vi "FOV_Zoom_Frame to Hex.vi"(8 "Objective":i8=20, 9 "Z pixel Size":i8=4, 11 "AOL_Globals":T1={"Imaging Protocol"=enum."AOL Z-Stack", "Number of POI"=0, "Number of Miniscans"=0, "Number of Trials"=0, "Number of Cycles "=0, "# Averaged Frames"=0, "Laser power (%)"=0, "Pockels (V)"=0.0, "Acquisition Length (sec)"=0.0, "Fill time (us)"=0.0, "POI Dwell time (us)"=0.0, "Miniscan Dwell time per pixel (us)"=0.0, "PMT 1"=0.0, "PMT 2"=0.0, "Back Apperture (mA)"=0.0, "Frame Size"=0, "Center Frequency"=0.0, "Field of View (norm)"=0.0, "DwellTime (us)"=0.0, "Wavelength (nm)"=0.0, "Zoom"=0.0, "AOL Z"=0.0, "AOL Mode"=enum."Raster", "GridXY"=0.0, "GridZ"=0.0, "TriggerPeriod (sec)"=0.0, "Number of Pixels in Miniscan"=0, "Experiment folder path"=path "", "X centre"=0.0, "Y centre"=0.0, "Angle (degrees)"=0.0, "Plane Mode"=0, "Threshold"=[], "Regenerate Chirps"=FALSE, "Rectangle ROI length (pixels)"=0, "Rectangle ROI height (pixels)"=0, "AOD fill"=4900, "StartupDelay"=0, "Samples Wait after Trigger"=5080, "Slip Cycle"=600000, "Add Cycle"=TRUE, "Functional Mode"=enum."Point", "Z Start"=0.0, "Z Stop"=0.0, "# Planes"=0} {"Plane Mode" items=["XY Plane", "XZ Plane", "YZ Plane", "arbitraryplane"]; "Frame Size" items=["100X100"=100, "128X128"=128, "200X200"=200, "256X256"=256, "512X512"=512, "1024x1024"=1024, "2048x2048"=2048]; "Back Apperture (mA)" format="%#.6g"; "Pockels (V)" format="%#.6g"; "PMT 2" format="%#.6g"; "PMT 1" format="%#.6g"; "Angle (degrees)" format="%#.6g"; "POI Dwell time (us)" format="%#.6g"}) -> (3 "FOV-Zoom-FrameSize Hex":string)   [LabVIEW 2017]
uses:
  Typedefs/Controls/AOL_Globals.ctl
  Typedefs/Imaging Protocols enum.ctl
  Typedefs/Frame Size.ctl
  Typedefs/AOL modes.ctl
  Typedefs/Plane Mode.ctl
  Typedefs/Functional Mode.ctl
  <vilib>/Utility/miscctls.llb/LVStringsAndValuesArrayTypeDef_SGL.ctl
panel:
  out "Field of view (um)":dbl
  # "SUBROUTINE"
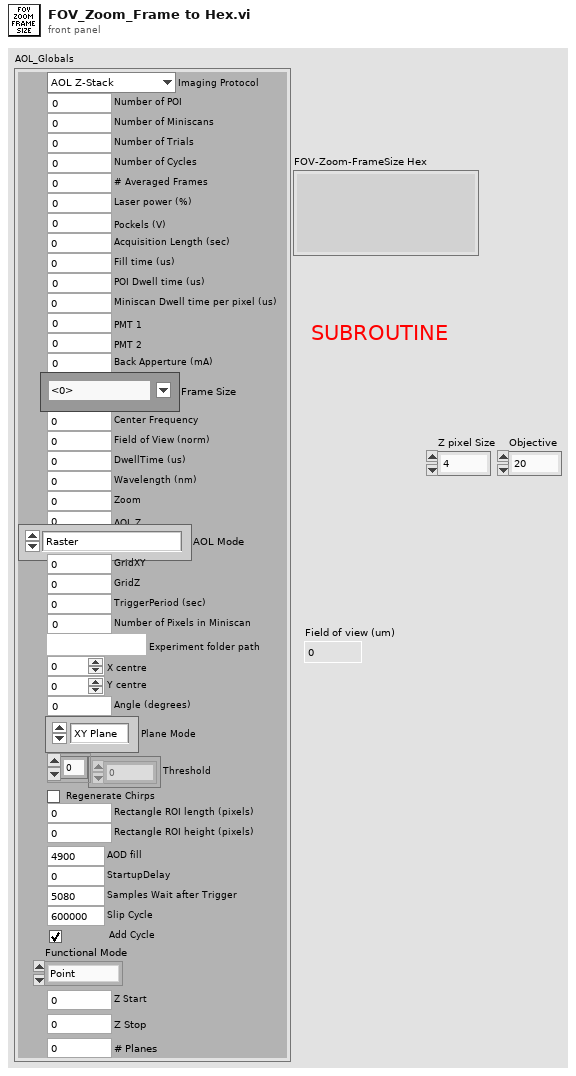
[diagram p1: front panel]
types:
  T1 = typedef "AOL_Globals.ctl" = cluster{"Imaging Protocol":T2, "Number of POI":u16, "Number of Miniscans":u16, "Number of Trials":u16, "Number of Cycles ":u64, "# Averaged Frames":u16, "Laser power (%)":u8, "Pockels (V)":dbl, "Acquisition Length (sec)":dbl, "Fill time (us)":dbl, "POI Dwell time (us)":dbl, "Miniscan Dwell time per pixel (us)":dbl, "PMT 1":dbl, "PMT 2":dbl, "Back Apperture (mA)":dbl, "Frame Size":T3, "Center Frequency":dbl, "Field of View (norm)":dbl, "DwellTime (us)":dbl, "Wavelength (nm)":dbl, "Zoom":dbl, "AOL Z":dbl, "AOL Mode":T4, "GridXY":dbl, "GridZ":dbl, "TriggerPeriod (sec)":dbl, "Number of Pixels in Miniscan":u16, "Experiment folder path":path, "X centre":dbl, "Y centre":dbl, "Angle (degrees)":dbl, "Plane Mode":T5, "Threshold":u16[], "Regenerate Chirps":bool, "Rectangle ROI length (pixels)":u16, "Rectangle ROI height (pixels)":u16, "AOD fill":u16, "StartupDelay":i32, "Samples Wait after Trigger":u16, "Slip Cycle":u32, "Add Cycle":bool, "Functional Mode":T6, "Z Start":dbl, "Z Stop":dbl, "# Planes":i32}
  T2 = typedef "Imaging Protocols enum.ctl" = enum16{"AOL Z-Stack", "Motor Z Stack", "Functional Acquisition", "Single Plane Acquisition", "Volume Acquisition", "Live Imaging", "Live Plane Imaging", "Live Volume Imaging"}
  T3 = typedef "Frame Size.ctl" = u16
  T4 = typedef "AOL modes.ctl" = enum16{"Raster", "Structural", "Pointing", "Mini Scan", "Alignment"}
  T5 = typedef "Plane Mode.ctl" = u16
  T6 = typedef "Functional Mode.ctl" = enum16{"Point", "Line", "Patch", "Plane", "Volume"}
  T7 = typedef "LVStringsAndValuesArrayTypeDef_SGL.ctl" = cluster{"String":string, "Value":sgl}[]
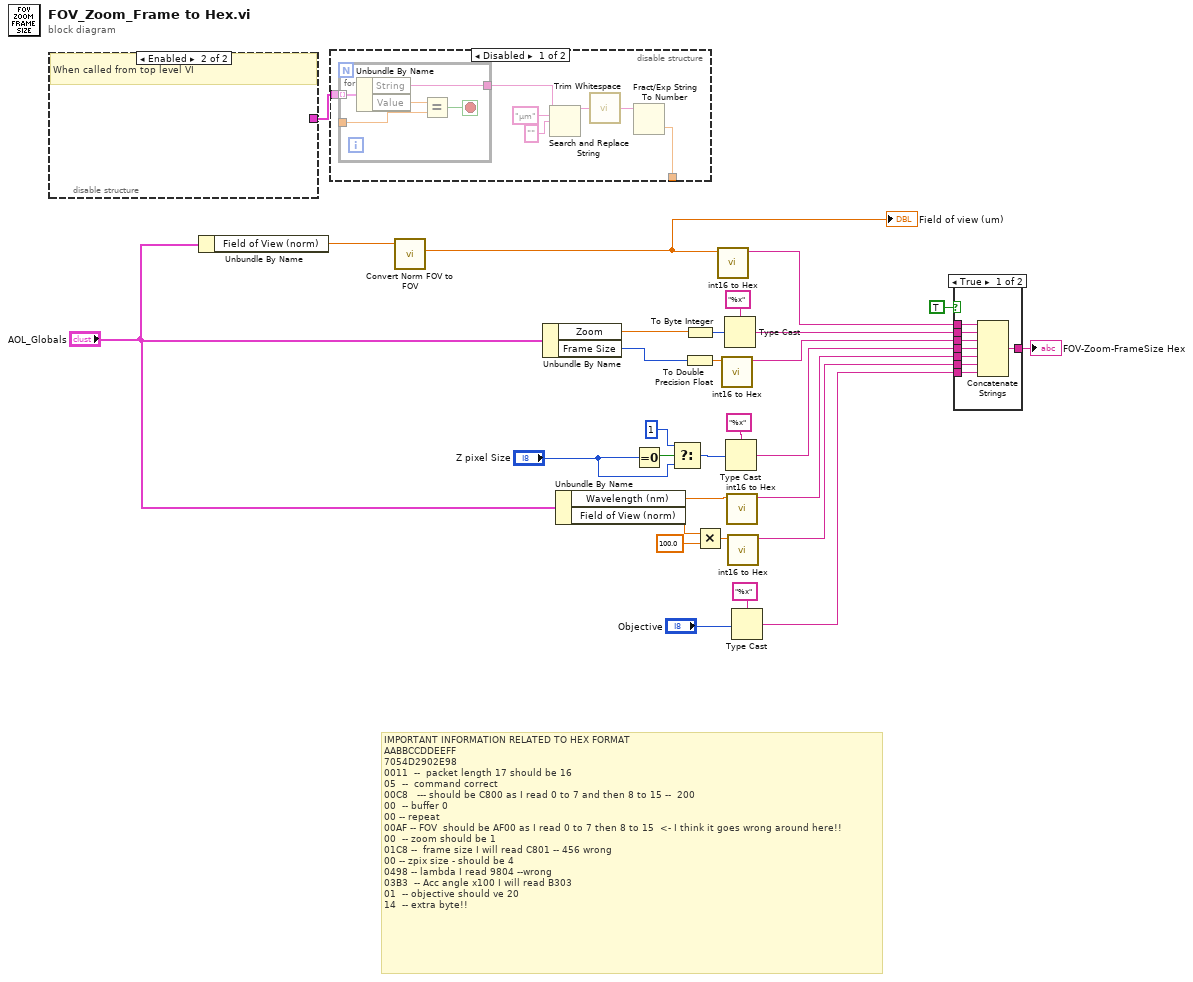
[diagram p0: block diagram]
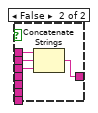
[diagram p3: hidden frame]
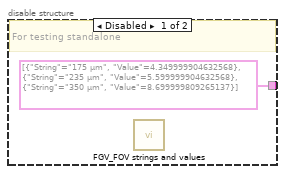
[diagram p4: hidden frame]
diagram:
  # "IMPORTANT INFORMATION RELATED TO HEX FORMAT\nAABBCCDDEEFF\n7054D2902E98\n0011  --  packet length 17 should be 16\n05  --  command correct\n00C8   --- should be C800 as I read 0 to 7 and then 8 to 15 --  200\n00  -- buffer 0\n00 -- repeat\n00AF -- FOV  should be AF00 as I read 0 to 7 then 8 to 15  <- I think it goes wrong around here!!\n00  -- zoom should be 1\n01C8 --  frame size I will read C801 -- 456 wrong\n00 -- zpix size - should be 4\n0498 -- lambda I read 9804 --wrong\n03B3  -- Acc angle x100 I will read B303\n01  -- objective should ve 20\n14  -- extra byte!!"
  n1 = disable-structure shown="Enabled" {
    disable-tunnel: [T7 [{"String"="175 µm", "Value"=4.35}, {"String"="235 µm", "Value"=5.6}, {"String"="350 µm", "Value"=8.7}] ("Strings And Values []") _] -> w20
    frame Disabled {
      # "For testing standalone"
      n2 = call "FGV_FOV strings and values.vi"() -> ()  [unwired: 10 in, 2 out]
    }
    frame Enabled {
      # "When called from top level VI"
    }
  }
  n3 = Unbundle By Name("AOL_Globals") -> ("Field of View (norm)"=w2:dbl)
  n4 = disable-structure shown="Disabled" {
    disable-tunnel: [w32 _] -> _
    disable-tunnel: w20 -> [w31 _]
    frame Disabled {
      n5 = for {
        tunnel: _ -> [w40]
        tunnel: w31 -> [w42] mode=indexing
        tunnel: [w38] -> w33
        stop <- w39 stop-if-true
        n6 = Unbundle By Name(w42) -> ("String"=w38:string, "Value"=w41:sgl)
        n7 = Equal?(x=w41, y=w40) -> (x = y?=w39:bool)
      }
      n8 = Search and Replace String(input string=w33, search string="µm", replace string="" ("replace string (\"\")")) -> (result string=w36:string)  [unwired: 5 in, 3 out]
      n9 = call <vilib>:"Trim Whitespace.vi"("string"=w36) -> ("trimmed string"=w37:string)  [unwired: 1 in]
      n10 = Fract/Exp String To Number(string=w37) -> (number=w32:dbl)  [unwired: 3 in, 1 out]
    }
    frame Enabled {
    }
  }
  n11 = call "Convert Norm FOV to FOV.vi"("Field of View(norm)"=w2) -> ("FOV"=w1:dbl)  [unwired: 9 in, 1 out]
  "Field of view (um)" <- w1
  n12 = Unbundle By Name("AOL_Globals") -> ("Zoom"=w25:dbl, "Frame Size"=w29:T3)
  n13 = Unbundle By Name("AOL_Globals") -> ("Wavelength (nm)"=w19:dbl, "Field of View (norm)"=w17:dbl)
  n14 = Equal To 0?(x="Z pixel Size") -> (x = 0?=w4:bool)
  n15 = Select(t=i8 1, s=w4, f="Z pixel Size") -> (s? t:f=w5:i8)
  n16 = To Byte Integer(number=w25) -> (8bit integer=w26:i8)
  n17 = To Double Precision Float(number=w29) -> (double precision float=w28:dbl)
  n18 = Multiply(x=w17, y=100.0) -> (x*y=w18:dbl)
  n19 = call "int16 to Hex.vi"("number"=w1) -> ("Hex string"=w24:string)  [unwired: 10 in]
  n20 = call "int16 to Hex.vi"("number"=w28) -> ("Hex string"=w22:string)  [unwired: 10 in]
  n21 = Type Cast(type="%x", x=w26) -> (*(type *) &x=w23:string)
  n22 = Type Cast(type="%x", x=w5) -> (*(type *) &x=w12:string)
  n23 = call "int16 to Hex.vi"("number"=w19) -> ("Hex string"=w11:string)  [unwired: 10 in]
  n24 = call "int16 to Hex.vi"("number"=w18) -> ("Hex string"=w10:string)  [unwired: 10 in]
  n25 = Type Cast(type="%x", x="Objective") -> (*(type *) &x=w9:string)
  n26 = case shown="True" TRUE {
    tunnel: w24 -> [w50 w54]
    tunnel: w23 -> [w49 w53]
    tunnel: w22 -> [w48 w52]
    tunnel: [w47 w51] -> w21
    tunnel: w12 -> [w46 _]
    tunnel: w11 -> [w45 _]
    tunnel: w10 -> [w44 _]
    tunnel: w9 -> [w43 _]
    frame True {
      n27 = Concatenate Strings(w50, w49, w48, w46, w45, w44, w43) -> (w47:string)
    }
    frame False {
      n28 = Concatenate Strings(w54, w53, w52) -> (w51:string)
    }
  }
  "FOV-Zoom-FrameSize Hex" <- w21
